vi "Save_Source_Type.vi"(8 "error in (no error)":errorcluster, 9 "index":i32, 10 "buildObject":T1, 11 "AB_Source in":refnum<class "AB_Source.lvclass">) -> (0 "error out":errorcluster, 3 "AB_Source out":refnum<class "AB_Source.lvclass">)   [LabVIEW 2020, in "AB_Source.lvclass"]
uses:
  <vilib>/AppBuilder/AB_Classes/Source/AB_Source.lvclass
  <resource>/Framework/Providers/API/ItemRef.ctl
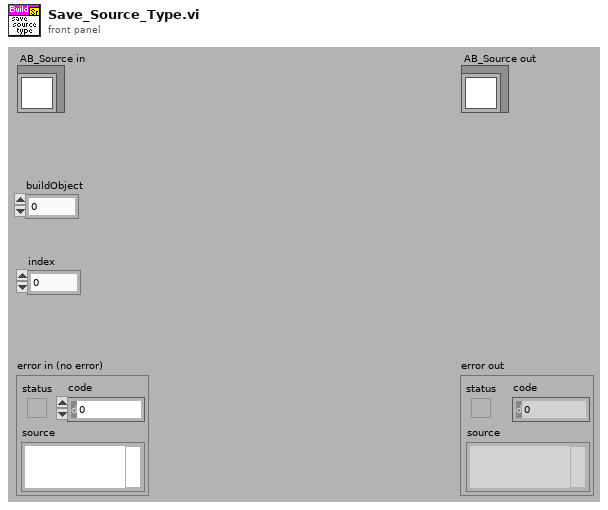
[diagram p1: front panel]
types:
  T1 = typedef "ItemRef.ctl" = u64
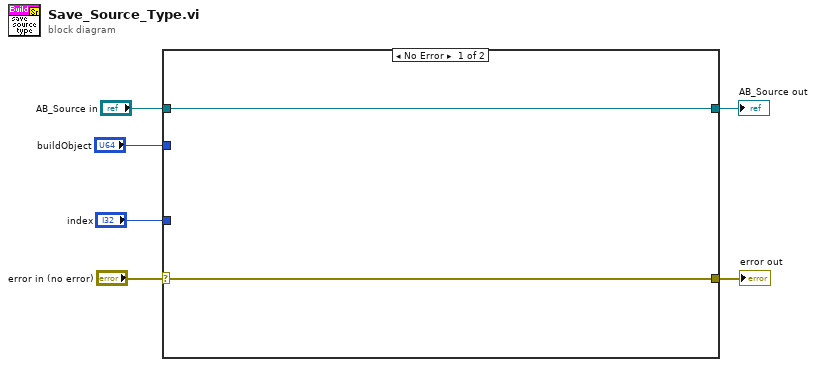
[diagram p0: block diagram]
diagram:
  n1 = case shown="No Error" "error in (no error)" {
    selector: "error in (no error)" -> [w7 w10]
    tunnel: [w7 w10] -> w5
    tunnel: [w8 w9] -> w3
    tunnel: "AB_Source in" -> [w8 w9]
    tunnel: "index" -> [_ _]
    tunnel: "buildObject" -> [_ _]
    frame No Error {
    }
    frame Error {
    }
  }
  "error out" <- w5
  "AB_Source out" <- w3
